vi "ELVIS III v1.0 Get Board Information.vi"(8 "error in":errorcluster) -> (0 "error out":errorcluster, 3 "Board Information":string)   [LabVIEW 2021]
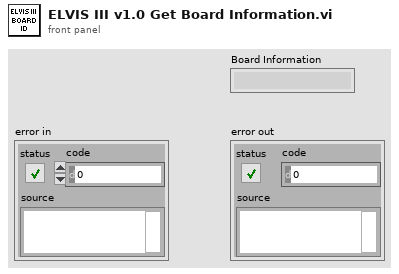
[diagram p1: front panel]
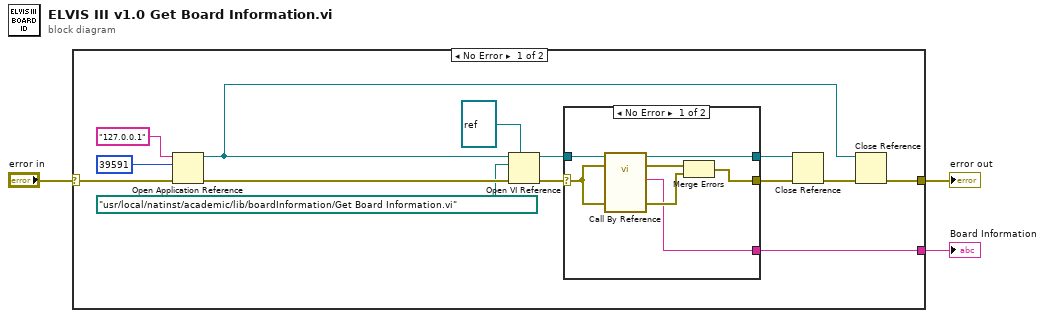
[diagram p0: block diagram]
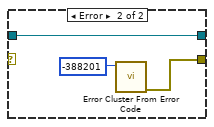
[diagram p2: hidden frame]
diagram:
  n1 = case shown="No Error" "error in" {
    selector: "error in" -> [w4 w28]
    tunnel: [w17 w28] -> w3
    tunnel: [w5 _] -> w2
    frame No Error {
      n2 = Open Application Reference(8:w4, 10:u16 39591 ("port number or service name (3363)"), 11:"127.0.0.1" ("Server IP")) -> (0:w16:errorcluster, 3:w15:refnum<vi>)  [unwired: 1 in]
      n3 = Open VI Reference(type specifier VI Refnum (for type only)=refnum<vi> refnum, application reference (local)=w15, vi path=path "/usr/local/natinst/academic/lib/boardInformation/Get Board Information.vi", error in (no error)=w16) -> (vi reference=w9:refnum<vi>, error out=w10:errorcluster)  [unwired: 2 in]
      n4 = case shown="No Error" w10 {
        selector: w10 -> [w18 _]
        tunnel: [w21 w26] -> w6
        tunnel: w9 -> [w24 w25]
        tunnel: [w20 w25] -> w14
        tunnel: [w19 _] -> w5
        frame No Error {
          n5 = call-by-ref "?"(reference=w24, error in=w18, 8:"error in (no error)"=w18) -> (reference out=w20:refnum<vi>, error out=w23:errorcluster, 0:"error out"=w22:errorcluster, "Board Information"=w19:string)  [unwired: 9 in]
          n6 = Merge Errors(w23, w22) -> (w21:errorcluster)
        }
        frame Error {
          n7 = call <vilib>:"Error Cluster From Error Code.vi"("error code (0)"=-388201) -> ("error out"=w26:errorcluster)  [unwired: 8 in]
        }
      }
      n8 = Close Reference(reference=w14, error in (no error)=w6) -> (error out=w7:errorcluster)
      n9 = Close Reference(reference=w15, error in (no error)=w7) -> (error out=w17:errorcluster)
    }
    frame Error {
    }
  }
  "error out" <- w3
  "Board Information" <- w2
